vi "AccX_new.vi"() -> ()   [LabVIEW 2019]
uses:
  DiscLevels.ctl
  #typedef_states.ctl
  <vilib>/rvi/Emulation/niFpgaGetClockAttributes.vi
  <vilib>/rvi/Emulation/niFpgaSctlEmulationGetInTimedLoop.vi
  <vilib>/rvi/Emulation/niFpgaEmulationReportErrorSimple.vi
  <vilib>/rvi/eio/common/nirviEmuTemplateMethod_errors.vi
  <vilib>/rvi/Emulation/niFpgaEmulationIsFPGAContextNoSignature.vi
  <vilib>/rvi/DataTransferAndStorage/Container/Common/niFpgaContainerGetUniqueNameForEmu.vi
  <vilib>/rvi/Memory/Memory_Emulation/niFpgaMemoryEmulationCacheClearOnFirstRun.vi
  <vilib>/rvi/Memory/Memory_Emulation/nirvimemoryEmulationManagerCache_MakeExclusive.vi
  <vilib>/rvi/Memory/Memory_Emulation/niFpgaMemoryEmulationValidateCache.vi
  <vilib>/rvi/Memory/Memory_Emulation/nirvimemoryEmulationManagerCache_InsertValue.vi
  <vilib>/Utility/error.llb/Clear Errors.vi
  <vilib>/rvi/Memory/Memory_Emulation/nirvimemoryEmulationManagerCache_ReleaseExclusive.vi
  <vilib>/rvi/Memory/Memory_Emulation/nirvimemoryEmulationManagerCache_GetValue.vi
  <vilib>/rvi/Memory/Memory_Emulation/nirvimemoryEmulationManagerCache_SetValue.vi
  <vilib>/rvi/Emulation/niFpgaProcessEmulError.vi
  <vilib>/rvi/Memory/Memory_Emulation/nirvimemoryFastEmulation.vi
  <vilib>/rvi/Memory/Memory_Emulation/nirvimemoryEmulation.vi
  <vilib>/rvi/errors/nirviReportUnexpectedCaseInternalError (U32).vi
  <vilib>/rvi/errors/niFpgaSetErrorForExecOnDevCompSimple.vi
  <vilib>/rvi/eio/common/nirviEmuReportErrorAndStop.vi
  <vilib>/rvi/FIFO/Fifo_Resource/nirvififoEmulationSetSize.vi
  <vilib>/rvi/FIFO/Fifo_Resource/nirviFifoEmulationQueueMgr.vi
  <instcachedir>/0/nirviFifoEmulationQueueMgr_E5CAEC123FF24DC58D834DCA3CDAA9B5.lvgen/nirviFifoEmulationQueueMgr_E5CAEC123FF24DC58D834DCA3CDAA9B5_001.vi
  <vilib>/rvi/FIFO/Fifo_Resource/nirvififoEmulationDetermineInputValidOut.vi
  <vilib>/rvi/FIFO/Fifo_Resource/nirvififoEmulationCreateLock.vi
  <vilib>/rvi/FIFO/Fifo_Resource/nirvififoEmulationObtainLock.vi
  <vilib>/rvi/FIFO/Fifo_Resource/nirvififoEmulationReleaseLock.vi
  <vilib>/rvi/occurrence/nirviWaitOnOccurrenceBase.vi
  <vilib>/rvi/errors/nirviReportUnexpectedCaseInternalError.vi
  <vilib>/rvi/Emulation/niFpgaCriticalErrorInLSC.vi
  <vilib>/rvi/interface/RandomDataEmulation/niFpgaRandomDataHandleErrors.vi
  <vilib>/eio/EIONode/EIONode.xnode
  <vilib>/rvi/DataTransferAndStorage/Container/XNode/niFpgaContainer.xnode
  <vilib>/rvi/DataTransferAndStorage/Register/Emulation/niFpgaRegisterEmulation.vi
  <vilib>/rvi/FIFO/Fifo_Resource/nirvififoEmulationWrite.vi
  <vilib>/rvi/interface/RandomDataEmulation/nirviRandomDataFpgaReadWriteTemplate.vi
  <vilib>/rvi/FIFO/Fifo_Resource/nirvififoEmulationRead.vi
panel:
  in  "Discrimination levels":T1
  in  "Samples amount":i16
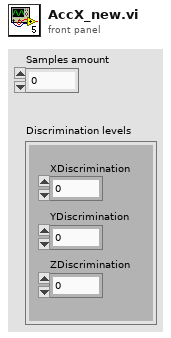
[diagram p1: front panel]
types:
  T1 = typedef "DiscLevels.ctl" = cluster{"XDiscrimination":i16, "YDiscrimination":i16, "ZDiscrimination":i16}
  T2 = typedef "#typedef_states.ctl" = enum16{"Wait", "Pretrigger", "Posttrigger"}
  T3 = cluster{"XDiscrimination":i16, "YDiscrimination":i16, "ZDiscrimination":i16}
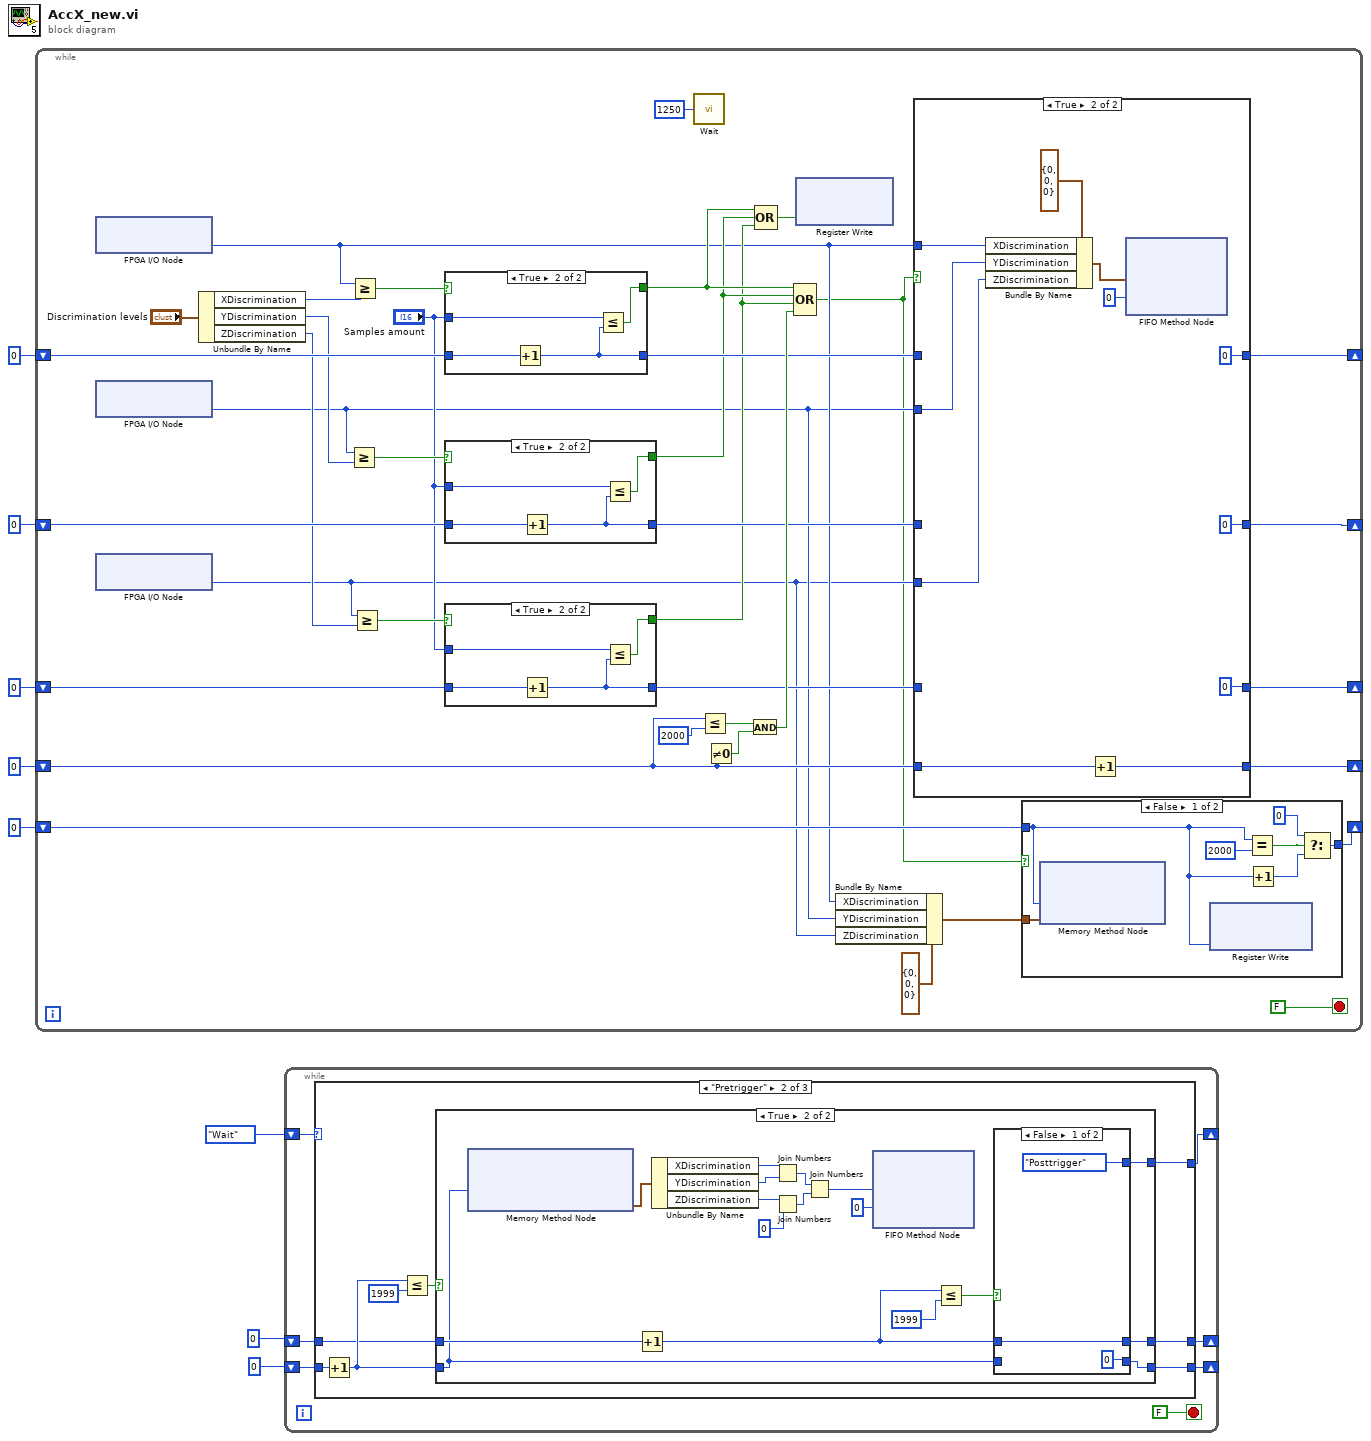
[diagram p0: block diagram]
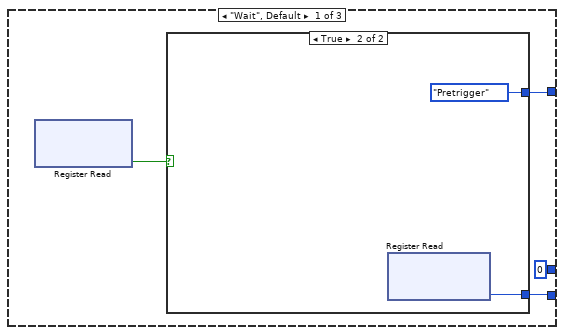
[diagram p2: hidden frame]
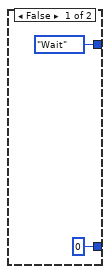
[diagram p3: hidden frame]
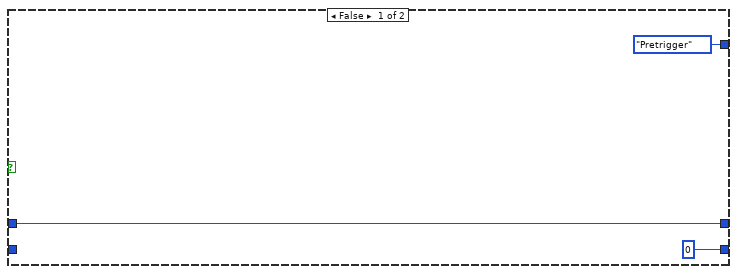
[diagram p4: hidden frame]
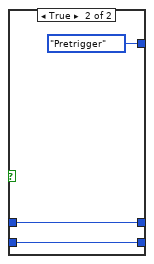
[diagram p5: hidden frame]
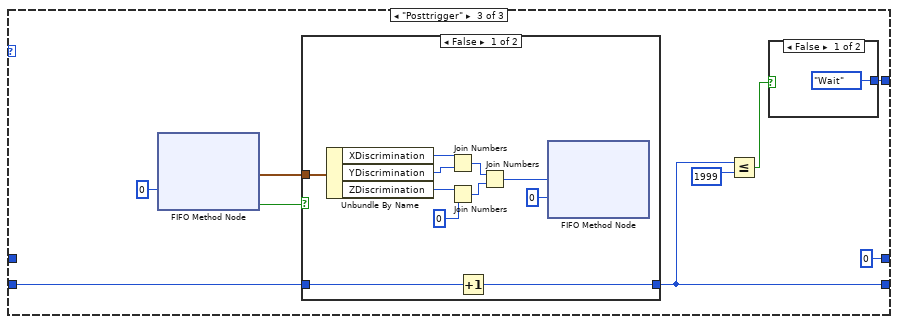
[diagram p6: hidden frame]
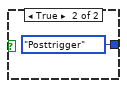
[diagram p7: hidden frame]
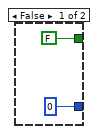
[diagram p10: hidden frame]
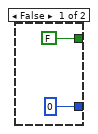
[diagram p11: hidden frame]
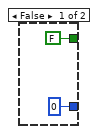
[diagram p12: hidden frame]
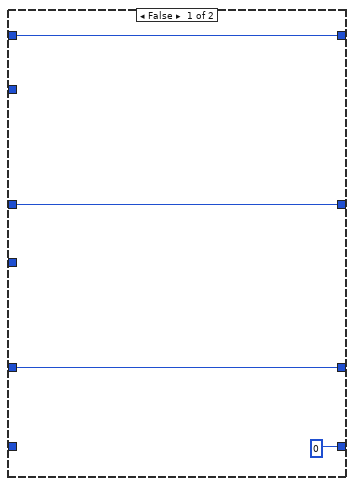
[diagram p13: hidden frame]
diagram:
  n1 = while {
    shift-right: [w45] -> _
    shift-left: i16 0 -> [w25]
    shift-right: [w38] -> _
    shift-left: i16 0 -> [w39]
    shift-right: [w32] -> _
    shift-left: i16 0 -> [w33]
    shift-right: [w26] -> _
    shift-left: i16 0 -> [w28]
    shift-right: [w18] -> _
    shift-left: u32 0 -> [w19]
    stop <- FALSE ("y") stop-if-true
    n2 = xnode "FPGA I/O Node"() -> ("AccelerationX"=w14:i16)  [unwired: 1 in, 1 out]
    n3 = xnode "FPGA I/O Node"() -> ("AccelerationY"=w13:i16)  [unwired: 1 in, 1 out]
    n4 = xnode "FPGA I/O Node"() -> ("AccelerationZ"=w12:i16)  [unwired: 1 in, 1 out]
    n5 = Unbundle By Name("Discrimination levels") -> ("XDiscrimination"=w36:i16, "YDiscrimination"=w34:i16, "ZDiscrimination"=w30:i16)
    n6 = Greater Or Equal?(x=w13, y=w34) -> (x >= y?=w35:bool)
    n7 = Greater Or Equal?(x=w14, y=w36) -> (x >= y?=w40:bool)
    n8 = Greater Or Equal?(x=w12, y=w30) -> (x >= y?=w31:bool)
    n9 = case shown="True" w40 {
      tunnel: w39 -> [_ w71]
      tunnel: [i16 0 w70] -> w22
      tunnel: [FALSE w69] -> w17
      tunnel: "Samples amount" -> [_ w68]
      frame False {
      }
      frame True {
        n10 = Increment(x=w71) -> (x+1=w70:i16)
        n11 = Less Or Equal?(x=w68, y=w70) -> (x <= y?=w69:bool)
      }
    }
    n12 = case shown="True" w35 {
      tunnel: w33 -> [_ w65]
      tunnel: [i16 0 w64] -> w21
      tunnel: [FALSE w63] -> w16
      tunnel: "Samples amount" -> [_ w62]
      frame False {
      }
      frame True {
        n13 = Increment(x=w65) -> (x+1=w64:i16)
        n14 = Less Or Equal?(x=w62, y=w64) -> (x <= y?=w63:bool)
      }
    }
    n15 = case shown="True" w31 {
      tunnel: w28 -> [_ w59]
      tunnel: [i16 0 w58] -> w20
      tunnel: [FALSE w57] -> w15
      tunnel: "Samples amount" -> [_ w56]
      frame False {
      }
      frame True {
        n16 = Increment(x=w59) -> (x+1=w58:i16)
        n17 = Less Or Equal?(x=w56, y=w58) -> (x <= y?=w57:bool)
      }
    }
    n18 = call "Wait"("Count(uSec)"=u32 1250) -> ()  [unwired: 1 out]
    n19 = Less Or Equal?(x=w25, y=i16 2000) -> (x <= y?=w43:bool)
    n20 = Not Equal To 0?(x=w25) -> (x != 0?=w42:bool)
    n21 = And(x=w43, y=w42) -> (x .and. y?=w27:bool)
    n22 = Compound Arithmetic op=OR(w17, w16, w15) -> (w10:bool)
    n23 = Compound Arithmetic op=OR(w17, w16, w15, w27) -> (w9:bool)
    n24 = xnode ("Register Write")("Data"=w10) -> ()  [unwired: 1 in, 1 out]
    n25 = Bundle By Name(cluster=T3 {"XDiscrimination"=0, "YDiscrimination"=0, "ZDiscrimination"=0} ("Data"), "XDiscrimination"=w14, "YDiscrimination"=w13, "ZDiscrimination"=w12) -> (w24:T3)
    n26 = case shown="True" w9 {
      tunnel: w14 -> [_ w80]
      tunnel: w25 -> [_ w86]
      tunnel: [i16 0 w85] -> w45
      tunnel: [w74 i16 0] -> w38
      tunnel: w22 -> [w74 _]
      tunnel: w13 -> [_ w79]
      tunnel: [w73 i16 0] -> w32
      tunnel: w21 -> [w73 _]
      tunnel: w12 -> [_ w78]
      tunnel: w20 -> [w72 _]
      tunnel: [w72 i16 0] -> w26
      frame False {
      }
      frame True {
        n27 = Bundle By Name(cluster=T3 {"XDiscrimination"=0, "YDiscrimination"=0, "ZDiscrimination"=0} ("Element"), "XDiscrimination"=w80, "YDiscrimination"=w79, "ZDiscrimination"=w78) -> (w76:T3)
        n28 = Increment(x=w86) -> (x+1=w85:i16)
        n29 = xnode ("FIFO Method Node")("Element"=w76, "Timeout"=0) -> ()  [unwired: 1 in, 2 out]
      }
    }
    n30 = case shown="False" w9 {
      tunnel: w24 -> [w52 _]
      tunnel: w19 -> [w47 w53]
      tunnel: [w46 w53] -> w18
      frame False {
        n31 = xnode ("Memory Method Node")("Address"=w47, "Data"=w52) -> ()  [unwired: 1 in, 1 out]
        n32 = xnode ("Register Write")("Data"=w47) -> ()  [unwired: 1 in, 1 out]
        n33 = Equal?(x=w47, y=u32 2000) -> (x = y?=w50:bool)
        n34 = Increment(x=w47) -> (x+1=w48:u32)
        n35 = Select(t=u32 0 ("f"), s=w50, f=w48) -> (s? t:f=w46:u32)
      }
      frame True {
      }
    }
  }
  n36 = while {
    shift-right: [w89] -> _
    shift-left: #typedef_states."Wait" ("States") -> [w92]
    shift-right: [w90] -> _
    shift-left: u32 0 -> [w91]
    shift-right: [w87] -> _
    shift-left: u32 0 -> [w88]
    stop <- FALSE stop-if-true
    n37 = case shown="\"Pretrigger\"" w92 {
      tunnel: w91 -> [_ w109 w141]
      tunnel: [w96 w106 w140] -> w90
      tunnel: [w95 w104 w137] -> w89
      tunnel: w88 -> [_ w103 _]
      tunnel: [u32 0 w102 u32 0] -> w87
      frame "Wait", Default {
        n38 = xnode ("Register Read")() -> ("Data"=w97:bool)  [unwired: 1 in, 1 out]
        n39 = case shown="True" w97 {
          tunnel: [u32 0 ("Data") w101] -> w96
          tunnel: [#typedef_states."Wait" ("States") #typedef_states."Pretrigger" ("States")] -> w95
          frame False {
          }
          frame True {
            n40 = xnode ("Register Read")() -> ("Data"=w101:u32)  [unwired: 1 in, 1 out]
          }
        }
      }
      frame "Pretrigger" {
        n41 = Increment(x=w109) -> (x+1=w105:u32)
        n42 = Less Or Equal?(x=w105, y=u32 1999) -> (x <= y?=w107:bool)
        n43 = case shown="True" w107 {
          tunnel: [u32 0 ("Data") w113] -> w106
          tunnel: w105 -> [_ w114]
          tunnel: [#typedef_states."Pretrigger" ("States") w128] -> w104
          tunnel: w103 -> [w110 w126]
          tunnel: [w110 w115] -> w102
          frame False {
          }
          frame True {
            n44 = xnode ("Memory Method Node")("Address"=w114) -> ("Data"=w117:T3)  [unwired: 1 in, 1 out]
            n45 = Increment(x=w126) -> (x+1=w116:u32)
            n46 = Unbundle By Name(w117) -> ("XDiscrimination"=w124:i16, "YDiscrimination"=w123:i16, "ZDiscrimination"=w122:i16)
            n47 = Join Numbers(hi=w124, lo=w123) -> ((hi.lo)=w119:u32)
            n48 = Join Numbers(hi=w122, lo=i16 0) -> ((hi.lo)=w120:u32)
            n49 = Join Numbers(hi=w119, lo=w120) -> ((hi.lo)=w118:u64)
            n50 = xnode ("FIFO Method Node")("Element"=w118, "Timeout"=0) -> ()  [unwired: 1 in, 2 out]
            n51 = Less Or Equal?(x=w116, y=u32 1999) -> (x <= y?=w129:bool)
            n52 = case shown="False" w129 {
              tunnel: [#typedef_states."Posttrigger" ("States") #typedef_states."Pretrigger" ("States")] -> w128
              tunnel: w116 -> [w131 w134]
              tunnel: [w131 w134] -> w115
              tunnel: w114 -> [_ w133]
              tunnel: [u32 0 w133] -> w113
              frame False {
              }
              frame True {
              }
            }
          }
        }
      }
      frame "Posttrigger" {
        n53 = xnode ("FIFO Method Node")("Timeout"=0) -> ("Element"=w144:T3, "Timed Out?"=w142:bool)  [unwired: 1 in, 1 out]
        n54 = case shown="False" w142 {
          tunnel: w144 -> [w156 _]
          tunnel: w141 -> [w148 w158]
          tunnel: [w147 w158] -> w140
          frame False {
            n55 = Unbundle By Name(w156) -> ("XDiscrimination"=w155:i16, "YDiscrimination"=w154:i16, "ZDiscrimination"=w153:i16)
            n56 = Join Numbers(hi=w155, lo=w154) -> ((hi.lo)=w150:u32)
            n57 = Join Numbers(hi=w153, lo=i16 0) -> ((hi.lo)=w151:u32)
            n58 = Increment(x=w148) -> (x+1=w147:u32)
            n59 = Join Numbers(hi=w150, lo=w151) -> ((hi.lo)=w149:u64)
            n60 = xnode ("FIFO Method Node")("Element"=w149, "Timeout"=0) -> ()  [unwired: 1 in, 2 out]
          }
          frame True {
          }
        }
        n61 = Less Or Equal?(x=w140, y=u32 1999) -> (x <= y?=w138:bool)
        n62 = case shown="False" w138 {
          tunnel: [#typedef_states."Wait" ("States") #typedef_states."Posttrigger" ("States")] -> w137
          frame False {
          }
          frame True {
          }
        }
      }
    }
  }
